vi "ief_send_command.vi"(0 "Tagprefix in":refnum<k21>, 3 "Command datum of type real":bool, 5 "Command datum":sgl format="%.2f", 7 "Command parameter":u16 format="%.0x", 9 "Command code":u16=6433 format="%.0x", 11 "error in (no error)":errorcluster, 12 "time out [s]":dbl=10.0 format="%.2f") -> (4 "Tagprefix out":refnum<k21>, 6 "Command error":bool, 8 "Command Error Code":u32, 10 "Command executed":bool, 14 "Command recognized":bool, 15 "error out (no error)":errorcluster)   [LabVIEW 2015, in "IEF Werner.lvlib"]
doc: "This VI sends a command to the IEF controller. Note that the tags of the DSC engine used by this VI have a strict name convention. This convention is described in the documentation of the VI tree.\n\nLicense Agreement for this software:\n\nCopyright (C)\nGesellschaft für Schwerionenforschung, GSI\nPlanckstr. 1\n64291 Darmstadt\nGermany\n\nContact: D.Beck@gsi.de \n\nThis program is free software; you can redistribute it and/or modify it under the terms of the \nGNU General Public License as published by the Free Software Foundation; either version 2 of \nthe license, or (at your option) any later version.\n\nThis program is distributed in the hope that it will be useful, but WITHOUT ANY WARRANTY; \nwithout even the implied warranty of MERCHANTABILITY or FITNESS FOR A PARTICULAR PURPOSE. See \nthe GNU General License for more details (http://www.gnu.org).\n\nGesellschaft für Schwerionenforschung, GSI\nPlanckstr. 1, 64291 Darmstadt, Germany\nFor all questions and ideas contact: M.Richter@gsi.de, H.Brand@gsi.de or D.Beck@gsi.de.\nLast update: 20-DEC-2002"
uses:
  IEF Werner.lvlib
  Packages/CSPP_Core/Libraries/Base/FGV Action.ctl
  <vilib>/lvdsc/legacy/tag/legacy_Write_Tag_(analog)7x.vi
  Packages/CSPP_Core/Libraries/Base/CS++Base.lvlib
  <vilib>/lvdsc/legacy/tag/legacy_Read_Tag_(analog)7x.vi
panel:
  # "IEF Send Command"
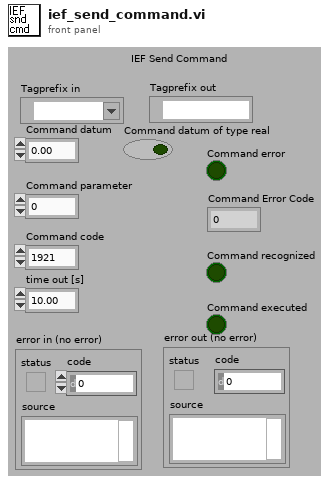
[diagram p1: front panel]
types:
  T1 = typedef "CS++Base.lvlib/FGV Action.ctl" = enum16{"add", "replace", "read", "remove", "reset", "get attributes"}
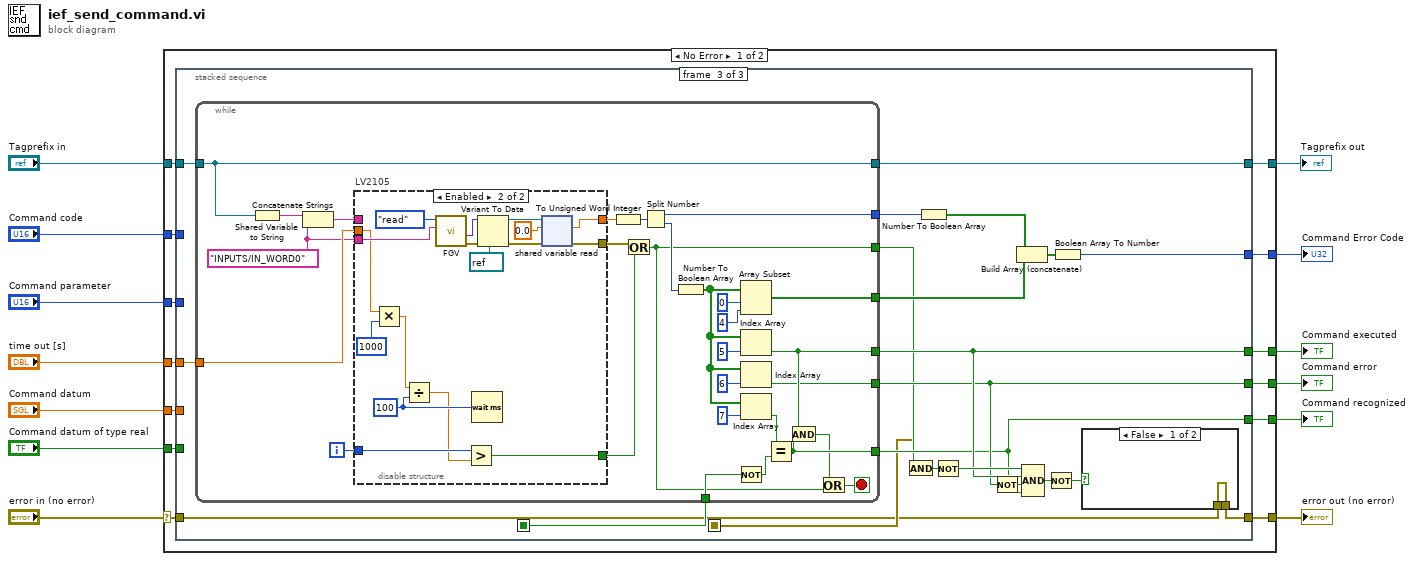
[diagram p0: block diagram]
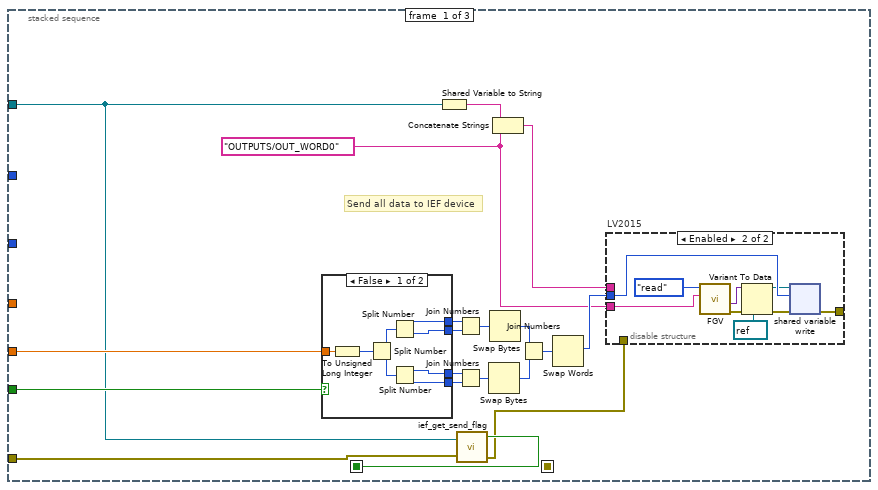
[diagram p2: hidden frame]
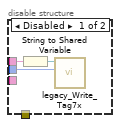
[diagram p3: hidden frame]
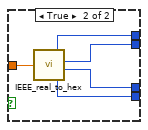
[diagram p4: hidden frame]
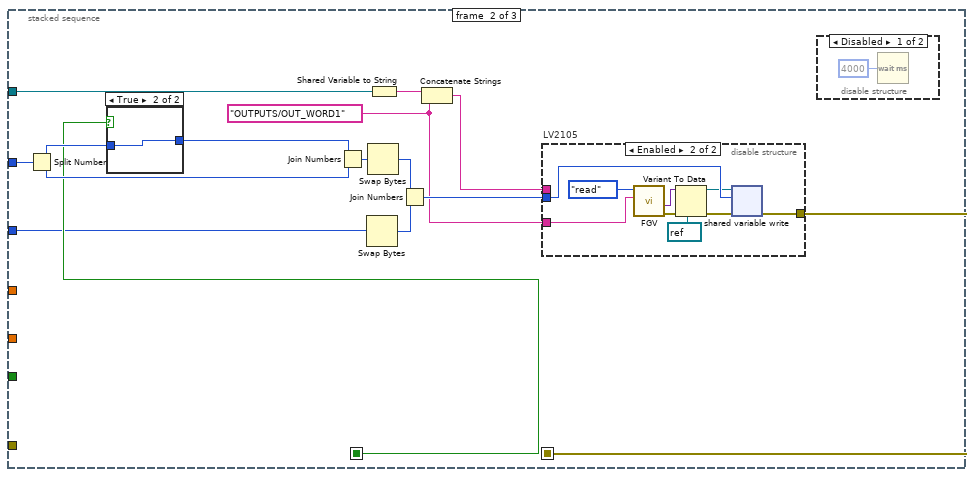
[diagram p5: hidden frame]
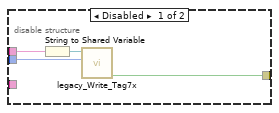
[diagram p7: hidden frame]
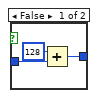
[diagram p8: hidden frame]
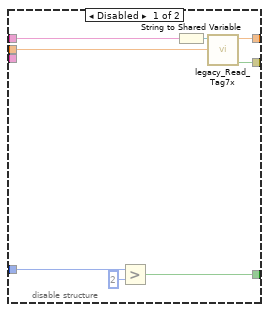
[diagram p9: hidden frame]
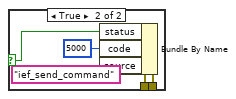
[diagram p10: hidden frame]
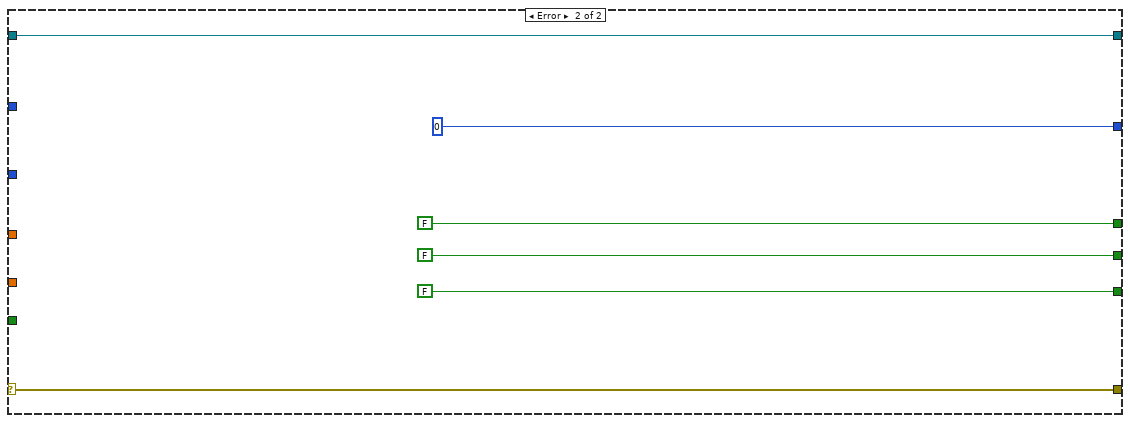
[diagram p11: hidden frame]
diagram:
  n1 = case shown="No Error" "error in (no error)" {
    selector: "error in (no error)" -> [w14 w184]
    tunnel: "Command datum" -> [w26 _]
    tunnel: "Command parameter" -> [w25 _]
    tunnel: "Command code" -> [w24 _]
    tunnel: [w23 FALSE] -> w11
    tunnel: [w22 FALSE] -> w10
    tunnel: [w21 FALSE] -> w9
    tunnel: [w20 u32 0] -> w8
    tunnel: "time out [s]" -> [w19 _]
    tunnel: "Command datum of type real" -> [w18 _]
    tunnel: [w17 w184] -> w4
    tunnel: "Tagprefix in" -> [w16 w189]
    tunnel: [w15 w189] -> w2
    frame No Error {
      n2 = stacked-sequence {
        seq-local: [w29 _ _] -> [_ w77 w113]
        seq-local: [_ w76 _] -> [_ _ w110]
        tunnel: w26 -> [w45 _ _]
        tunnel: w25 -> [_ w72 _]
        tunnel: w24 -> [_ w78 _]
        tunnel: [_ _ w115] -> w23
        tunnel: [_ _ w116] -> w22
        tunnel: [_ _ w117] -> w21
        tunnel: [_ _ w121] -> w20
        tunnel: w19 -> [_ _ w118]
        tunnel: w18 -> [w44 _ _]
        tunnel: w14 -> [w28 _ w109]
        tunnel: [_ _ w108] -> w17
        tunnel: w16 -> [w32 w74 w106]
        tunnel: [_ _ w105] -> w15
        frame #0 {
          w30 = "OUTPUTS/OUT_WORD0"
          # "Send all data to IEF device"
          n3 = case shown="False" w44 {
            tunnel: w45 -> [w65 w70]
            tunnel: [w61 w69] -> w42
            tunnel: [w60 w67] -> w41
            tunnel: [w59 w66] -> w40
            tunnel: [w58 w68] -> w39
            frame False {
              n4 = To Unsigned Long Integer(number=w65) -> (unsigned 32bit integer=w64:u32)
              n5 = Split Number(x=w64) -> (hi(x)=w63:u16, lo(x)=w62:u16)
              n6 = Split Number(x=w63) -> (hi(x)=w61:u8, lo(x)=w60:u8)
              n7 = Split Number(x=w62) -> (hi(x)=w59:u8, lo(x)=w58:u8)
            }
            frame True {
              n8 = call "IEEE_real_to_hex.vi"("number 5"=w70) -> ("number"=w69:u8, "number 2"=w67:u8, "number 3"=w66:u8, "number 4"=w68:u8)
            }
          }
          n9 = Shared Variable to String(1:w32) -> (0:w33:string)
          n10 = Join Numbers(hi=w42, lo=w41) -> ((hi.lo)=w38:u16)
          n11 = Join Numbers(hi=w40, lo=w39) -> ((hi.lo)=w37:u16)
          n12 = call "ief_get_send_flag.vi"("tag prefix in"=w32, "error in (no error)"=w28) -> ("Send-Flag"=w29:bool, "error out (no error)"=w27:errorcluster)  [unwired: 1 out]
          n13 = Swap Bytes(anything=w37) -> (byte swapped=w35:u16)
          n14 = Swap Bytes(anything=w38) -> (byte swapped=w36:u16)
          n15 = Concatenate Strings(w33, w30) -> (w31:string)
          n16 = Join Numbers(hi=w36, lo=w35) -> ((hi.lo)=w43:u32)
          n17 = Swap Words(1:w43) -> (0:w34:u32)
          n18 = disable-structure "LV2015" shown="Enabled" {
            disable-tunnel: w34 -> [w48 w57]
            disable-tunnel: w31 -> [w47 _]
            disable-tunnel: w30 -> [_ w50]
            disable-tunnel: [_ w49] -> _
            disable-tunnel: w27 -> [_ _]
            frame Disabled {
              n19 = String to Shared Variable(0:w47) -> (2:w46:refnum<k21>)  [unwired: 1 out]
              n20 = call-poly <vilib>:"legacy_Write_Tag7x.vi"("value"=w48, "tag name"=w46) -> ()  [unwired: 7 in, 3 out]
            }
            frame Enabled {
              n21 = call "FGV.vi"("Attribute Name"=w50, "Action (read)"=FGV_Action."read") -> ("Error Out"=w56:errorcluster, "Data out"=w55:variant)  [unwired: 5 in, 3 out]
              n22 = Variant To Data(error in=w56, type=refnum<k21> refnum ("shared variable refnum in"), Variant=w55) -> (data=w51:refnum<k21>, error out=w52:errorcluster)
              n23 = shared-variable-write(w51, w52, w57) -> (w49:errorcluster)  [unwired: 1 out]
            }
          }
        }
        frame #1 {
          w71 = "OUTPUTS/OUT_WORD1"
          n24 = Split Number(x=w78) -> (hi(x)=w79:u8, lo(x)=w85:u8)
          n25 = case shown="True" w77 {
            tunnel: w79 -> [w100 w103]
            tunnel: [w102 w103] -> w83
            frame False {
              n26 = Add(x=u8 128 ("y"), y=w100) -> (x+y=w102:u8)
            }
            frame True {
            }
          }
          n27 = Join Numbers(hi=w83, lo=w85) -> ((hi.lo)=w82:u16)
          n28 = Swap Bytes(anything=w72) -> (byte swapped=w80:u16)
          n29 = Swap Bytes(anything=w82) -> (byte swapped=w81:u16)
          n30 = Shared Variable to String(1:w74) -> (0:w75:string)
          n31 = Join Numbers(hi=w81, lo=w80) -> ((hi.lo)=w84:u32)
          n32 = Concatenate Strings(w75, w71) -> (w73:string)
          n33 = disable-structure "LV2105" shown="Enabled" {
            disable-tunnel: w84 -> [w90 w99]
            disable-tunnel: [w89 w98] -> w76
            disable-tunnel: w73 -> [w88 _]
            disable-tunnel: w71 -> [_ w91]
            frame Disabled {
              n34 = String to Shared Variable(0:w88) -> (2:w87:refnum<k21>)  [unwired: 1 out]
              n35 = call-poly <vilib>:"legacy_Write_Tag7x.vi"("value"=w90, "tag name"=w87) -> ("error"=w89:bool)  [unwired: 7 in, 2 out]
            }
            frame Enabled {
              n36 = call "FGV.vi"("Attribute Name"=w91, "Action (read)"=FGV_Action."read") -> ("Error Out"=w97:errorcluster, "Data out"=w96:variant)  [unwired: 5 in, 3 out]
              n37 = Variant To Data(error in=w97, type=refnum<k21> refnum ("shared variable refnum in"), Variant=w96) -> (data=w92:refnum<k21>, error out=w93:errorcluster)
              n38 = shared-variable-write(w92, w93, w99) -> (w98:errorcluster)  [unwired: 1 out]
            }
          }
          n39 = disable-structure shown="Disabled" {
            frame Disabled {
              n40 = Wait (ms)(milliseconds to wait=u32 4000) -> ()  [unwired: 1 out]
            }
            frame Enabled {
            }
          }
        }
        frame #2 {
          n41 = while {
            tunnel: [w133] -> w105
            tunnel: w106 -> [w133]
            tunnel: [w152] -> w123
            tunnel: w118 -> [w136]
            tunnel: [w151] -> w117
            tunnel: [w150] -> w116
            tunnel: [w149] -> w115
            tunnel: w113 -> [w148]
            tunnel: [w147] -> w112
            tunnel: [w128] -> w111
            i -> [w126]
            stop <- w131 stop-if-true
            w127 = "INPUTS/IN_WORD0" ("string")
            n42 = Shared Variable to String(1:w133) -> (0:w135:string)
            n43 = Concatenate Strings(w135, w127) -> (w134:string)
            n44 = disable-structure "LV2105" shown="Enabled" {
              disable-tunnel: [w160 w176] -> w139
              disable-tunnel: w136 -> [w159 w163]
              disable-tunnel: w134 -> [w158 _]
              disable-tunnel: [w156 w175] -> w129
              disable-tunnel: w127 -> [_ w168]
              disable-tunnel: w126 -> [w154 w167]
              disable-tunnel: [w153 w166] -> w125
              frame Disabled {
                n45 = Greater?(x=w154, y=2) -> (0:w153:bool)
                n46 = String to Shared Variable(0:w158) -> (2:w157:refnum<k21>)  [unwired: 1 out]
                n47 = call-poly <vilib>:"legacy_Read_Tag7x.vi"("timeout (secs) (0)"=w159, "tag name"=w157) -> ("error"=w156:bool, "value"=w160:dbl)  [unwired: 3 in, 5 out]
              }
              frame Enabled {
                w165 = u32 100 ("milliseconds to wait")
                n48 = Multiply(x=w163, y=u32 1000 ("milliseconds to wait")) -> (x*y=w162:dbl)
                n49 = Divide(x=w162, y=w165) -> (x/y=w164:dbl)
                n50 = call "FGV.vi"("Attribute Name"=w168, "Action (read)"=FGV_Action."read") -> ("Error Out"=w174:errorcluster, "Data out"=w173:variant)  [unwired: 5 in, 3 out]
                n51 = Greater?(x=w167, y=w164) -> (0:w166:bool)
                n52 = Wait (ms)(milliseconds to wait=w165) -> ()  [unwired: 1 out]
                n53 = Variant To Data(error in=w174, type=refnum<k21> refnum ("shared variable refnum in"), Variant=w173) -> (data=w170:refnum<k21>, error out=w171:errorcluster)
                n54 = shared-variable-read(w170, w171, 0.0) -> (w175:errorcluster, w176:dbl)  [unwired: 2 out]
              }
            }
            n55 = To Unsigned Word Integer(number=w139) -> (unsigned 16bit integer=w130:u16)
            n56 = Or(x=w129, y=w125) -> (x .or. y?=w128:bool)
            n57 = Split Number(x=w130) -> (hi(x)=w147:u8, lo(x)=w137:u8)
            n58 = Number To Boolean Array(number=w137) -> (Boolean array=w143:bool[])
            n59 = Not(x=w148) -> (.not. x?=w138:bool)
            n60 = Array Subset(array=w143, index=0 ("Index"), length=4 ("Index")) -> (w152:bool[])
            n61 = Index Array(array=w143, index=5 ("Index")) -> (element=w151:bool)
            n62 = Index Array(array=w143, index=6 ("Index")) -> (element=w150:bool)
            n63 = Index Array(array=w143, index=7 ("Index")) -> (element=w140:bool)
            n64 = Equal?(x=w140, y=w138) -> (x = y?=w149:bool)
            n65 = And(x=w151, y=w149) -> (x .and. y?=w132:bool)
            n66 = Or(x=w132, y=w128) -> (x .or. y?=w131:bool)
          }
          n67 = And(x=w110, y=w111) -> (x .and. y?=w120:bool)
          n68 = Number To Boolean Array(number=w112) -> (Boolean array=w124:bool[])
          n69 = Not(x=w120) -> (.not. x?=w119:bool)
          n70 = Not(x=w116) -> (.not. x?=w114:bool)
          n71 = Build Array (concatenate)(w124, w123) -> (w122:bool[])
          n72 = Compound Arithmetic op=AND(w119, w117, w114, w115) -> (w107:bool)
          n73 = Not(x=w107) -> (.not. x?=w104:bool)
          n74 = Boolean Array To Number(Boolean array=w122) -> (number=w121:u32)
          n75 = case shown="False" w104 {
            selector: w104 -> [_ w181]
            tunnel: w109 -> [w178 w183]
            tunnel: [w178 w182] -> w108
            frame False {
            }
            frame True {
              n76 = Bundle By Name(cluster=w183, "status"=w181, "code"=5000, "source"="ief_send_command") -> (w182:errorcluster)
            }
          }
        }
      }
    }
    frame Error {
    }
  }
  "Command recognized" <- w11
  "Command error" <- w10
  "Command executed" <- w9
  "Command Error Code" <- w8
  "error out (no error)" <- w4
  "Tagprefix out" <- w2
